vi "syndrom(4800).vi"(7 "Кадр для  вычисления \nсиндрома":bool[](array[boolean])) -> (8 "Синдром":bool[](array[boolean]))   [LabVIEW 2013]
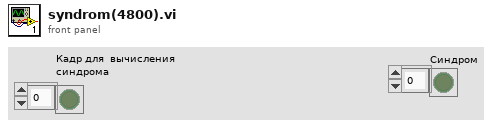
[diagram p1: front panel]
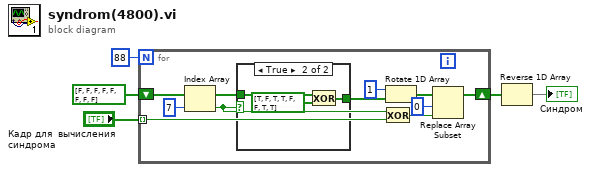
[diagram p0: block diagram]
diagram:
  n1 = for {
    N: 88 -> [_]
    tunnel: "Кадр для  вычисления \nсиндрома" -> [w6] mode=indexing
    shift-right: [w10] -> w3
    shift-left: bool[] [FALSE, FALSE, FALSE, FALSE, FALSE, FALSE, FALSE, FALSE] -> [w14]
    n2 = Index Array(array=w14, index=7) -> (element=w7:bool)
    n3 = case shown="True" w7 {
      tunnel: w14 -> [w16 w19]
      tunnel: [w16 w18] -> w13
      frame False {
      }
      frame True {
        n4 = Exclusive Or(1:bool[] [TRUE, FALSE, TRUE, TRUE, FALSE, FALSE, TRUE, TRUE] ("y"), 2:w19) -> (0:w18:bool[])
      }
    }
    n5 = Exclusive Or(1:w6, 2:w7) -> (0:w8:bool)
    n6 = Rotate 1D Array(1:w13, 2:1 ("n")) -> (0:w11:bool[])
    n7 = Replace Array Subset(array=w11, new element=w8, index=0) -> (w10:bool[])
  }
  n8 = Reverse 1D Array(array=w3) -> (reversed array=→"Синдром":bool[])
